vi "DDS_Clock.vi"() -> ()   [LabVIEW 2016] (continued)
{"total time[ms]"=82.69999999999744, "f1 [Hz] CH0"=310800000.00000006}, {"total time[ms]"=82.74999999999744, "f1 [Hz] CH0"=311000000.0}, {"total time[ms]"=82.74999999999744, "f1 [Hz] CH0"=311000000.0}, {"total time[ms]"=82.79999999999744, "f1 [Hz] CH0"=311200000.00000006}, {"total time[ms]"=82.79999999999744, "f1 [Hz] CH0"=311200000.00000006}, {"total time[ms]"=82.84999999999744, "f1 [Hz] CH0"=311400000.00000006}, {"total time[ms]"=82.84999999999744, "f1 [Hz] CH0"=311400000.00000006}, {"total time[ms]"=82.89999999999743, "f1 [Hz] CH0"=311600000.00000006}, {"total time[ms]"=82.89999999999743, "f1 [Hz] CH0"=311600000.00000006}, {"total time[ms]"=82.94999999999743, "f1 [Hz] CH0"=311800000.0}, {"total time[ms]"=82.94999999999743, "f1 [Hz] CH0"=311800000.0}, {"total time[ms]"=82.99999999999743, "f1 [Hz] CH0"=312000000.0}, {"total time[ms]"=82.99999999999743, "f1 [Hz] CH0"=312000000.0}, {"total time[ms]"=83.04999999999742, "f1 [Hz] CH0"=312200000.00000006}, {"total time[ms]"=83.04999999999742, "f1 [Hz] CH0"=312200000.00000006}, {"total time[ms]"=83.09999999999742, "f1 [Hz] CH0"=312400000.0}, {"total time[ms]"=83.09999999999742, "f1 [Hz] CH0"=312400000.0}, {"total time[ms]"=83.14999999999742, "f1 [Hz] CH0"=312600000.00000006}, {"total time[ms]"=83.14999999999742, "f1 [Hz] CH0"=312600000.00000006}, {"total time[ms]"=83.19999999999742, "f1 [Hz] CH0"=312800000.0}, {"total time[ms]"=83.19999999999742, "f1 [Hz] CH0"=312800000.0}, {"total time[ms]"=83.24999999999741, "f1 [Hz] CH0"=313000000.00000006}, {"total time[ms]"=83.24999999999741, "f1 [Hz] CH0"=313000000.00000006}, {"total time[ms]"=83.29999999999741, "f1 [Hz] CH0"=313200000.00000006}, {"total time[ms]"=83.29999999999741, "f1 [Hz] CH0"=313200000.00000006}, {"total time[ms]"=83.34999999999741, "f1 [Hz] CH0"=313400000.00000006}, {"total time[ms]"=83.34999999999741, "f1 [Hz] CH0"=313400000.00000006}, {"total time[ms]"=83.3999999999974, "f1 [Hz] CH0"=313600000.00000006}, {"total time[ms]"=83.3999999999974, "f1 [Hz] CH0"=313600000.00000006}, {"total time[ms]"=83.4499999999974, "f1 [Hz] CH0"=313800000.0}, {"total time[ms]"=83.4499999999974, "f1 [Hz] CH0"=313800000.0}, {"total time[ms]"=83.4999999999974, "f1 [Hz] CH0"=314000000.0}, {"total time[ms]"=83.4999999999974, "f1 [Hz] CH0"=314000000.0}, {"total time[ms]"=83.5499999999974, "f1 [Hz] CH0"=314200000.00000006}, {"total time[ms]"=83.5499999999974, "f1 [Hz] CH0"=314200000.00000006}, {"total time[ms]"=83.5999999999974, "f1 [Hz] CH0"=314400000.00000006}, {"total time[ms]"=83.5999999999974, "f1 [Hz] CH0"=314400000.00000006}, {"total time[ms]"=83.64999999999739, "f1 [Hz] CH0"=314600000.0}, {"total time[ms]"=83.64999999999739, "f1 [Hz] CH0"=314600000.0}, {"total time[ms]"=83.69999999999739, "f1 [Hz] CH0"=314800000.00000006}, {"total time[ms]"=83.69999999999739, "f1 [Hz] CH0"=314800000.00000006}, {"total time[ms]"=83.74999999999739, "f1 [Hz] CH0"=315000000.0}, {"total time[ms]"=83.74999999999739, "f1 [Hz] CH0"=315000000.0}, {"total time[ms]"=83.79999999999738, "f1 [Hz] CH0"=315200000.00000006}, {"total time[ms]"=83.79999999999738, "f1 [Hz] CH0"=315200000.00000006}, {"total time[ms]"=83.84999999999738, "f1 [Hz] CH0"=315400000.00000006}, {"total time[ms]"=83.84999999999738, "f1 [Hz] CH0"=315400000.00000006}, {"total time[ms]"=83.89999999999738, "f1 [Hz] CH0"=315600000.0}, {"total time[ms]"=83.89999999999738, "f1 [Hz] CH0"=315600000.0}, {"total time[ms]"=83.94999999999737, "f1 [Hz] CH0"=315800000.00000006}, {"total time[ms]"=83.94999999999737, "f1 [Hz] CH0"=315800000.00000006}, {"total time[ms]"=83.99999999999737, "f1 [Hz] CH0"=316000000.0}, {"total time[ms]"=83.99999999999737, "f1 [Hz] CH0"=316000000.0}, {"total time[ms]"=84.04999999999737, "f1 [Hz] CH0"=316200000.00000006}, {"total time[ms]"=84.04999999999737, "f1 [Hz] CH0"=316200000.00000006}, {"total time[ms]"=84.09999999999737, "f1 [Hz] CH0"=316400000.00000006}, {"total time[ms]"=84.09999999999737, "f1 [Hz] CH0"=316400000.00000006}, {"total time[ms]"=84.14999999999736, "f1 [Hz] CH0"=316600000.00000006}, {"total time[ms]"=84.14999999999736, "f1 [Hz] CH0"=316600000.00000006}, {"total time[ms]"=84.19999999999736, "f1 [Hz] CH0"=316800000.0}, {"total time[ms]"=84.19999999999736, "f1 [Hz] CH0"=316800000.0}, {"total time[ms]"=84.24999999999736, "f1 [Hz] CH0"=317000000.0}, {"total time[ms]"=84.24999999999736, "f1 [Hz] CH0"=317000000.0}, {"total time[ms]"=84.29999999999735, "f1 [Hz] CH0"=317200000.00000006}, {"total time[ms]"=84.29999999999735, "f1 [Hz] CH0"=317200000.00000006}, {"total time[ms]"=84.34999999999735, "f1 [Hz] CH0"=317400000.0}, {"total time[ms]"=84.34999999999735, "f1 [Hz] CH0"=317400000.0}, {"total time[ms]"=84.39999999999735, "f1 [Hz] CH0"=317600000.00000006}, {"total time[ms]"=84.39999999999735, "f1 [Hz] CH0"=317600000.00000006}, {"total time[ms]"=84.44999999999735, "f1 [Hz] CH0"=317800000.0}, {"total time[ms]"=84.44999999999735, "f1 [Hz] CH0"=317800000.0}, {"total time[ms]"=84.49999999999734, "f1 [Hz] CH0"=318000000.00000006}, {"total time[ms]"=84.49999999999734, "f1 [Hz] CH0"=318000000.00000006}, {"total time[ms]"=84.54999999999734, "f1 [Hz] CH0"=318200000.00000006}, {"total time[ms]"=84.54999999999734, "f1 [Hz] CH0"=318200000.00000006}, {"total time[ms]"=84.59999999999734, "f1 [Hz] CH0"=318400000.00000006}, {"total time[ms]"=84.59999999999734, "f1 [Hz] CH0"=318400000.00000006}, {"total time[ms]"=84.64999999999733, "f1 [Hz] CH0"=318600000.00000006}, {"total time[ms]"=84.64999999999733, "f1 [Hz] CH0"=318600000.00000006}, {"total time[ms]"=84.69999999999733, "f1 [Hz] CH0"=318800000.0}, {"total time[ms]"=84.69999999999733, "f1 [Hz] CH0"=318800000.0}, {"total time[ms]"=84.74999999999733, "f1 [Hz] CH0"=319000000.0}, {"total time[ms]"=84.74999999999733, "f1 [Hz] CH0"=319000000.0}, {"total time[ms]"=84.79999999999733, "f1 [Hz] CH0"=319200000.0000001}, {"total time[ms]"=84.79999999999733, "f1 [Hz] CH0"=319200000.0000001}, {"total time[ms]"=84.84999999999732, "f1 [Hz] CH0"=319400000.00000006}, {"total time[ms]"=84.84999999999732, "f1 [Hz] CH0"=319400000.00000006}, {"total time[ms]"=84.89999999999732, "f1 [Hz] CH0"=319600000.0}, {"total time[ms]"=84.89999999999732, "f1 [Hz] CH0"=319600000.0}, {"total time[ms]"=84.94999999999732, "f1 [Hz] CH0"=319800000.00000006}, {"total time[ms]"=84.94999999999732, "f1 [Hz] CH0"=319800000.00000006}, {"total time[ms]"=84.99999999999731, "f1 [Hz] CH0"=320000000.0}, {"total time[ms]"=84.99999999999731, "f1 [Hz] CH0"=320000000.0}, {"total time[ms]"=85.04999999999731, "f1 [Hz] CH0"=319800000.0}, {"total time[ms]"=85.04999999999731, "f1 [Hz] CH0"=319800000.0}, {"total time[ms]"=85.09999999999731, "f1 [Hz] CH0"=319599999.99999994}, {"total time[ms]"=85.09999999999731, "f1 [Hz] CH0"=319599999.99999994}, {"total time[ms]"=85.1499999999973, "f1 [Hz] CH0"=319400000.0}, {"total time[ms]"=85.1499999999973, "f1 [Hz] CH0"=319400000.0}, {"total time[ms]"=85.1999999999973, "f1 [Hz] CH0"=319199999.99999994}, {"total time[ms]"=85.1999999999973, "f1 [Hz] CH0"=319199999.99999994}, {"total time[ms]"=85.2499999999973, "f1 [Hz] CH0"=319000000.0}, {"total time[ms]"=85.2499999999973, "f1 [Hz] CH0"=319000000.0}, {"total time[ms]"=85.2999999999973, "f1 [Hz] CH0"=318799999.99999994}, {"total time[ms]"=85.2999999999973, "f1 [Hz] CH0"=318799999.99999994}, {"total time[ms]"=85.3499999999973, "f1 [Hz] CH0"=318599999.99999994}, {"total time[ms]"=85.3499999999973, "f1 [Hz] CH0"=318599999.99999994}, {"total time[ms]"=85.39999999999729, "f1 [Hz] CH0"=318399999.99999994}, {"total time[ms]"=85.39999999999729, "f1 [Hz] CH0"=318399999.99999994}, {"total time[ms]"=85.44999999999729, "f1 [Hz] CH0"=318200000.0}, {"total time[ms]"=85.44999999999729, "f1 [Hz] CH0"=318200000.0}, {"total time[ms]"=85.49999999999729, "f1 [Hz] CH0"=318000000.0}, {"total time[ms]"=85.49999999999729, "f1 [Hz] CH0"=318000000.0}, {"total time[ms]"=85.54999999999728, "f1 [Hz] CH0"=317799999.99999994}, {"total time[ms]"=85.54999999999728, "f1 [Hz] CH0"=317799999.99999994}, {"total time[ms]"=85.59999999999728, "f1 [Hz] CH0"=317600000.0}, {"total time[ms]"=85.59999999999728, "f1 [Hz] CH0"=317600000.0}, {"total time[ms]"=85.64999999999728, "f1 [Hz] CH0"=317399999.99999994}, {"total time[ms]"=85.64999999999728, "f1 [Hz] CH0"=317399999.99999994}, {"total time[ms]"=85.69999999999727, "f1 [Hz] CH0"=317200000.0}, {"total time[ms]"=85.69999999999727, "f1 [Hz] CH0"=317200000.0}, {"total time[ms]"=85.74999999999727, "f1 [Hz] CH0"=316999999.99999994}, {"total time[ms]"=85.74999999999727, "f1 [Hz] CH0"=316999999.99999994}, {"total time[ms]"=85.79999999999727, "f1 [Hz] CH0"=316799999.99999994}, {"total time[ms]"=85.79999999999727, "f1 [Hz] CH0"=316799999.99999994}, {"total time[ms]"=85.84999999999727, "f1 [Hz] CH0"=316599999.99999994}, {"total time[ms]"=85.84999999999727, "f1 [Hz] CH0"=316599999.99999994}, {"total time[ms]"=85.89999999999726, "f1 [Hz] CH0"=316399999.99999994}, {"total time[ms]"=85.89999999999726, "f1 [Hz] CH0"=316399999.99999994}, {"total time[ms]"=85.94999999999726, "f1 [Hz] CH0"=316200000.0}, {"total time[ms]"=85.94999999999726, "f1 [Hz] CH0"=316200000.0}, {"total time[ms]"=85.99999999999726, "f1 [Hz] CH0"=316000000.0}, {"total time[ms]"=85.99999999999726, "f1 [Hz] CH0"=316000000.0}, {"total time[ms]"=86.04999999999725, "f1 [Hz] CH0"=315799999.99999994}, {"total time[ms]"=86.04999999999725, "f1 [Hz] CH0"=315799999.99999994}, {"total time[ms]"=86.09999999999725, "f1 [Hz] CH0"=315599999.99999994}, {"total time[ms]"=86.09999999999725, "f1 [Hz] CH0"=315599999.99999994}, {"total time[ms]"=86.14999999999725, "f1 [Hz] CH0"=315400000.0}, {"total time[ms]"=86.14999999999725, "f1 [Hz] CH0"=315400000.0}, {"total time[ms]"=86.19999999999725, "f1 [Hz] CH0"=315199999.99999994}, {"total time[ms]"=86.19999999999725, "f1 [Hz] CH0"=315199999.99999994}, {"total time[ms]"=86.24999999999724, "f1 [Hz] CH0"=315000000.0}, {"total time[ms]"=86.24999999999724, "f1 [Hz] CH0"=315000000.0}, {"total time[ms]"=86.29999999999724, "f1 [Hz] CH0"=314799999.99999994}, {"total time[ms]"=86.29999999999724, "f1 [Hz] CH0"=314799999.99999994}, {"total time[ms]"=86.34999999999724, "f1 [Hz] CH0"=314599999.99999994}, {"total time[ms]"=86.34999999999724, "f1 [Hz] CH0"=314599999.99999994}, {"total time[ms]"=86.39999999999723, "f1 [Hz] CH0"=314400000.0}, {"total time[ms]"=86.39999999999723, "f1 [Hz] CH0"=314400000.0}, {"total time[ms]"=86.44999999999723, "f1 [Hz] CH0"=314199999.99999994}, {"total time[ms]"=86.44999999999723, "f1 [Hz] CH0"=314199999.99999994}, {"total time[ms]"=86.49999999999723, "f1 [Hz] CH0"=314000000.0}, {"total time[ms]"=86.49999999999723, "f1 [Hz] CH0"=314000000.0}, {"total time[ms]"=86.54999999999723, "f1 [Hz] CH0"=313799999.99999994}, {"total time[ms]"=86.54999999999723, "f1 [Hz] CH0"=313799999.99999994}, {"total time[ms]"=86.59999999999722, "f1 [Hz] CH0"=313599999.99999994}, {"total time[ms]"=86.59999999999722, "f1 [Hz] CH0"=313599999.99999994}, {"total time[ms]"=86.64999999999722, "f1 [Hz] CH0"=313399999.99999994}, {"total time[ms]"=86.64999999999722, "f1 [Hz] CH0"=313399999.99999994}, {"total time[ms]"=86.69999999999722, "f1 [Hz] CH0"=313200000.0}, {"total time[ms]"=86.69999999999722, "f1 [Hz] CH0"=313200000.0}, {"total time[ms]"=86.74999999999721, "f1 [Hz] CH0"=313000000.0}, {"total time[ms]"=86.74999999999721, "f1 [Hz] CH0"=313000000.0}, {"total time[ms]"=86.79999999999721, "f1 [Hz] CH0"=312799999.99999994}, {"total time[ms]"=86.79999999999721, "f1 [Hz] CH0"=312799999.99999994}, {"total time[ms]"=86.84999999999721, "f1 [Hz] CH0"=312600000.0}, {"total time[ms]"=86.84999999999721, "f1 [Hz] CH0"=312600000.0}, {"total time[ms]"=86.8999999999972, "f1 [Hz] CH0"=312399999.99999994}, {"total time[ms]"=86.8999999999972, "f1 [Hz] CH0"=312399999.99999994}, {"total time[ms]"=86.9499999999972, "f1 [Hz] CH0"=312200000.0}, {"total time[ms]"=86.9499999999972, "f1 [Hz] CH0"=312200000.0}, {"total time[ms]"=86.9999999999972, "f1 [Hz] CH0"=311999999.99999994}, {"total time[ms]"=86.9999999999972, "f1 [Hz] CH0"=311999999.99999994}, {"total time[ms]"=87.0499999999972, "f1 [Hz] CH0"=311799999.99999994}, {"total time[ms]"=87.0499999999972, "f1 [Hz] CH0"=311799999.99999994}, {"total time[ms]"=87.0999999999972, "f1 [Hz] CH0"=311599999.99999994}, {"total time[ms]"=87.0999999999972, "f1 [Hz] CH0"=311599999.99999994}, {"total time[ms]"=87.14999999999719, "f1 [Hz] CH0"=311399999.99999994}, {"total time[ms]"=87.14999999999719, "f1 [Hz] CH0"=311399999.99999994}, {"total time[ms]"=87.19999999999719, "f1 [Hz] CH0"=311200000.0}, {"total time[ms]"=87.19999999999719, "f1 [Hz] CH0"=311200000.0}, {"total time[ms]"=87.24999999999719, "f1 [Hz] CH0"=311000000.0}, {"total time[ms]"=87.24999999999719, "f1 [Hz] CH0"=311000000.0}, {"total time[ms]"=87.29999999999718, "f1 [Hz] CH0"=310799999.99999994}, {"total time[ms]"=87.29999999999718, "f1 [Hz] CH0"=310799999.99999994}, {"total time[ms]"=87.34999999999718, "f1 [Hz] CH0"=310599999.99999994}, {"total time[ms]"=87.34999999999718, "f1 [Hz] CH0"=310599999.99999994}, {"total time[ms]"=87.39999999999718, "f1 [Hz] CH0"=310400000.0}, {"total time[ms]"=87.39999999999718, "f1 [Hz] CH0"=310400000.0}, {"total time[ms]"=87.44999999999717, "f1 [Hz] CH0"=310199999.99999994}, {"total time[ms]"=87.44999999999717, "f1 [Hz] CH0"=310199999.99999994}, {"total time[ms]"=87.49999999999717, "f1 [Hz] CH0"=310000000.0}, {"total time[ms]"=87.49999999999717, "f1 [Hz] CH0"=310000000.0}, {"total time[ms]"=87.54999999999717, "f1 [Hz] CH0"=309799999.99999994}, {"total time[ms]"=87.54999999999717, "f1 [Hz] CH0"=309799999.99999994}, {"total time[ms]"=87.59999999999717, "f1 [Hz] CH0"=309599999.99999994}, {"total time[ms]"=87.59999999999717, "f1 [Hz] CH0"=309599999.99999994}, {"total time[ms]"=87.64999999999716, "f1 [Hz] CH0"=309400000.0}, {"total time[ms]"=87.64999999999716, "f1 [Hz] CH0"=309400000.0}, {"total time[ms]"=87.69999999999716, "f1 [Hz] CH0"=309199999.99999994}, {"total time[ms]"=87.69999999999716, "f1 [Hz] CH0"=309199999.99999994}, {"total time[ms]"=87.74999999999716, "f1 [Hz] CH0"=309000000.0}, {"total time[ms]"=87.74999999999716, "f1 [Hz] CH0"=309000000.0}, {"total time[ms]"=87.79999999999715, "f1 [Hz] CH0"=308799999.99999994}, {"total time[ms]"=87.79999999999715, "f1 [Hz] CH0"=308799999.99999994}, {"total time[ms]"=87.84999999999715, "f1 [Hz] CH0"=308599999.99999994}, {"total time[ms]"=87.84999999999715, "f1 [Hz] CH0"=308599999.99999994}, {"total time[ms]"=87.89999999999715, "f1 [Hz] CH0"=308399999.99999994}, {"total time[ms]"=87.89999999999715, "f1 [Hz] CH0"=308399999.99999994}, {"total time[ms]"=87.94999999999715, "f1 [Hz] CH0"=308200000.0}, {"total time[ms]"=87.94999999999715, "f1 [Hz] CH0"=308200000.0}, {"total time[ms]"=87.99999999999714, "f1 [Hz] CH0"=308000000.0}, {"total time[ms]"=87.99999999999714, "f1 [Hz] CH0"=308000000.0}, {"total time[ms]"=88.04999999999714, "f1 [Hz] CH0"=307799999.99999994}, {"total time[ms]"=88.04999999999714, "f1 [Hz] CH0"=307799999.99999994}, {"total time[ms]"=88.09999999999714, "f1 [Hz] CH0"=307600000.0}, {"total time[ms]"=88.09999999999714, "f1 [Hz] CH0"=307600000.0}, {"total time[ms]"=88.14999999999714, "f1 [Hz] CH0"=307399999.99999994}, {"total time[ms]"=88.14999999999714, "f1 [Hz] CH0"=307399999.99999994}, {"total time[ms]"=88.19999999999713, "f1 [Hz] CH0"=307200000.0}, {"total time[ms]"=88.19999999999713, "f1 [Hz] CH0"=307200000.0}, {"total time[ms]"=88.24999999999713, "f1 [Hz] CH0"=306999999.99999994}, {"total time[ms]"=88.24999999999713, "f1 [Hz] CH0"=306999999.99999994}, {"total time[ms]"=88.29999999999713, "f1 [Hz] CH0"=306799999.99999994}, {"total time[ms]"=88.29999999999713, "f1 [Hz] CH0"=306799999.99999994}, {"total time[ms]"=88.34999999999712, "f1 [Hz] CH0"=306599999.99999994}, {"total time[ms]"=88.34999999999712, "f1 [Hz] CH0"=306599999.99999994}, {"total time[ms]"=88.39999999999712, "f1 [Hz] CH0"=306399999.99999994}, {"total time[ms]"=88.39999999999712, "f1 [Hz] CH0"=306399999.99999994}, {"total time[ms]"=88.44999999999712, "f1 [Hz] CH0"=306200000.0}, {"total time[ms]"=88.44999999999712, "f1 [Hz] CH0"=306200000.0}, {"total time[ms]"=88.49999999999712, "f1 [Hz] CH0"=306000000.0}, {"total time[ms]"=88.49999999999712, "f1 [Hz] CH0"=306000000.0}, {"total time[ms]"=88.54999999999711, "f1 [Hz] CH0"=305799999.99999994}, {"total time[ms]"=88.54999999999711, "f1 [Hz] CH0"=305799999.99999994}, {"total time[ms]"=88.59999999999711, "f1 [Hz] CH0"=305599999.99999994}, {"total time[ms]"=88.59999999999711, "f1 [Hz] CH0"=305599999.99999994}, {"total time[ms]"=88.6499999999971, "f1 [Hz] CH0"=305400000.0}, {"total time[ms]"=88.6499999999971, "f1 [Hz] CH0"=305400000.0}, {"total time[ms]"=88.6999999999971, "f1 [Hz] CH0"=305199999.99999994}, {"total time[ms]"=88.6999999999971, "f1 [Hz] CH0"=305199999.99999994}, {"total time[ms]"=88.7499999999971, "f1 [Hz] CH0"=305000000.0}, {"total time[ms]"=88.7499999999971, "f1 [Hz] CH0"=305000000.0}, {"total time[ms]"=88.7999999999971, "f1 [Hz] CH0"=304799999.99999994}, {"total time[ms]"=88.7999999999971, "f1 [Hz] CH0"=304799999.99999994}, {"total time[ms]"=88.8499999999971, "f1 [Hz] CH0"=304599999.99999994}, {"total time[ms]"=88.8499999999971, "f1 [Hz] CH0"=304599999.99999994}, {"total time[ms]"=88.89999999999709, "f1 [Hz] CH0"=304400000.0}, {"total time[ms]"=88.89999999999709, "f1 [Hz] CH0"=304400000.0}, {"total time[ms]"=88.94999999999709, "f1 [Hz] CH0"=304199999.99999994}, {"total time[ms]"=88.94999999999709, "f1 [Hz] CH0"=304199999.99999994}, {"total time[ms]"=88.99999999999709, "f1 [Hz] CH0"=304000000.0}, {"total time[ms]"=88.99999999999709, "f1 [Hz] CH0"=304000000.0}, {"total time[ms]"=89.04999999999708, "f1 [Hz] CH0"=303799999.99999994}, {"total time[ms]"=89.04999999999708, "f1 [Hz] CH0"=303799999.99999994}, {"total time[ms]"=89.09999999999708, "f1 [Hz] CH0"=303599999.99999994}, {"total time[ms]"=89.09999999999708, "f1 [Hz] CH0"=303599999.99999994}, {"total time[ms]"=89.14999999999708, "f1 [Hz] CH0"=303399999.99999994}, {"total time[ms]"=89.14999999999708, "f1 [Hz] CH0"=303399999.99999994}, {"total time[ms]"=89.19999999999708, "f1 [Hz] CH0"=303200000.0}, {"total time[ms]"=89.19999999999708, "f1 [Hz] CH0"=303200000.0}, {"total time[ms]"=89.24999999999707, "f1 [Hz] CH0"=303000000.0}, {"total time[ms]"=89.24999999999707, "f1 [Hz] CH0"=303000000.0}, {"total time[ms]"=89.29999999999707, "f1 [Hz] CH0"=302799999.99999994}, {"total time[ms]"=89.29999999999707, "f1 [Hz] CH0"=302799999.99999994}, {"total time[ms]"=89.34999999999707, "f1 [Hz] CH0"=302600000.0}, {"total time[ms]"=89.34999999999707, "f1 [Hz] CH0"=302600000.0}, {"total time[ms]"=89.39999999999706, "f1 [Hz] CH0"=302399999.99999994}, {"total time[ms]"=89.39999999999706, "f1 [Hz] CH0"=302399999.99999994}, {"total time[ms]"=89.44999999999706, "f1 [Hz] CH0"=302200000.0}, {"total time[ms]"=89.44999999999706, "f1 [Hz] CH0"=302200000.0}, {"total time[ms]"=89.49999999999706, "f1 [Hz] CH0"=301999999.99999994}, {"total time[ms]"=89.49999999999706, "f1 [Hz] CH0"=301999999.99999994}, {"total time[ms]"=89.54999999999706, "f1 [Hz] CH0"=301799999.99999994}, {"total time[ms]"=89.54999999999706, "f1 [Hz] CH0"=301799999.99999994}, {"total time[ms]"=89.59999999999705, "f1 [Hz] CH0"=301599999.99999994}, {"total time[ms]"=89.59999999999705, "f1 [Hz] CH0"=301599999.99999994}, {"total time[ms]"=89.64999999999705, "f1 [Hz] CH0"=301399999.99999994}, {"total time[ms]"=89.64999999999705, "f1 [Hz] CH0"=301399999.99999994}, {"total time[ms]"=89.69999999999705, "f1 [Hz] CH0"=301200000.0}, {"total time[ms]"=89.69999999999705, "f1 [Hz] CH0"=301200000.0}, {"total time[ms]"=89.74999999999704, "f1 [Hz] CH0"=301000000.0}, {"total time[ms]"=89.74999999999704, "f1 [Hz] CH0"=301000000.0}, {"total time[ms]"=89.79999999999704, "f1 [Hz] CH0"=300799999.99999994}, {"total time[ms]"=89.79999999999704, "f1 [Hz] CH0"=300799999.99999994}, {"total time[ms]"=89.84999999999704, "f1 [Hz] CH0"=300599999.99999994}, {"total time[ms]"=89.84999999999704, "f1 [Hz] CH0"=300599999.99999994}, {"total time[ms]"=89.89999999999704, "f1 [Hz] CH0"=300400000.0}, {"total time[ms]"=89.89999999999704, "f1 [Hz] CH0"=300400000.0}, {"total time[ms]"=89.94999999999703, "f1
